vi "Move_mm.vi"(8 "error in":errorcluster, 10 "mm":dbl, 11 "connection ID":refnum<k5>) -> (0 "error out":errorcluster, 2 "Driver response":bool, 3 "TCP Network Connection out":refnum<k5>)   [LabVIEW 2019]
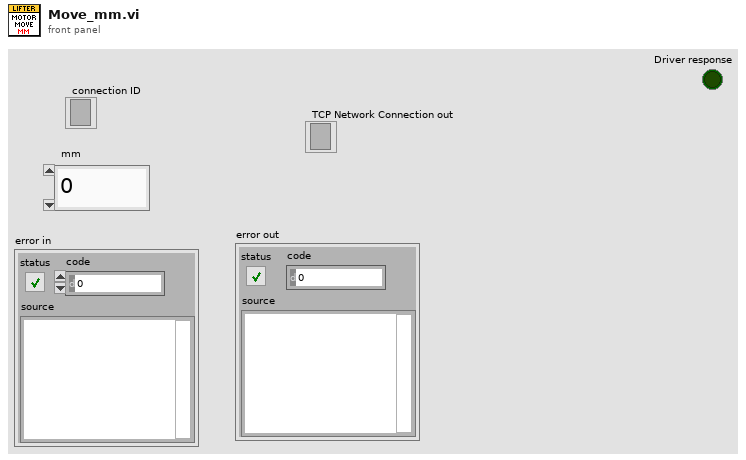
[diagram p1: front panel]
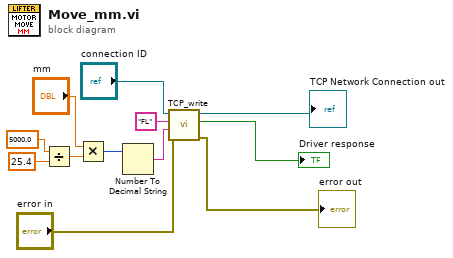
[diagram p0: block diagram]
diagram:
  n1 = Divide(x=5000.0, y=25.4) -> (x/y=w8:dbl)
  n2 = Multiply(x="mm", y=w8) -> (x*y=w9:i32)
  n3 = Number To Decimal String(number=w9) -> (decimal integer string=w10:string)  [unwired: 1 in]
  n4 = call "TCP_write.vi"("error in"="error in", "Parameter 2"=w10, "Parameter 1"="FL" ("string"), "connection ID"="connection ID") -> ("error out"=→"error out":errorcluster, "Driver response"=→"Driver response":bool, "TCP Network Connection out"=→"TCP Network Connection out":refnum<k5>)  [unwired: 5 in]
